vi "Render.vi"(9 "Size (1)":i32=1, 10 "Keys":map{string, string[]}(c390), 11 "Content in":string) -> (3 "Content out":string)   [LabVIEW 2021, in "HttpServer.lvlib"]
uses:
  HttpServer.lvlib
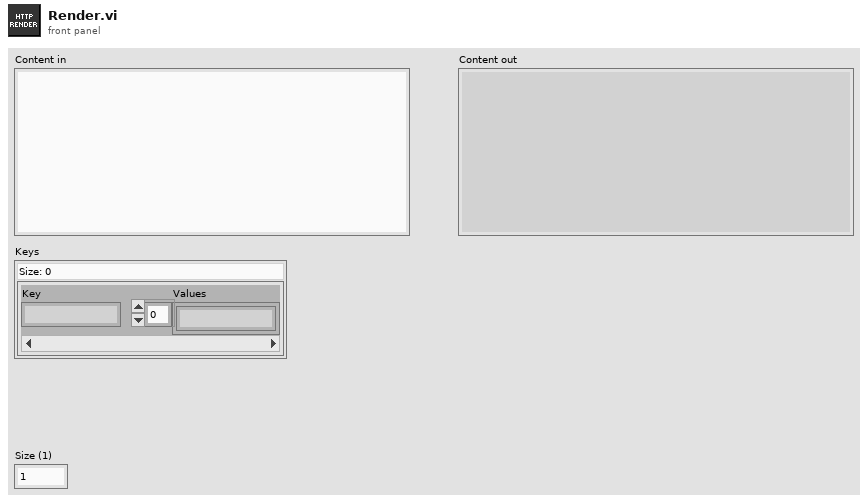
[diagram p1: front panel]
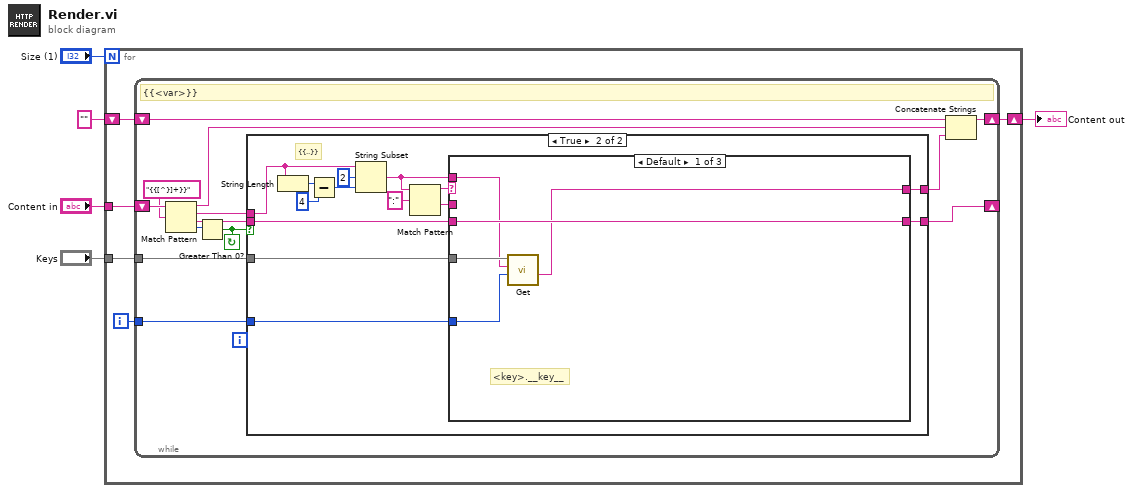
[diagram p0: block diagram]
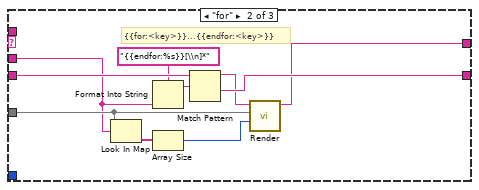
[diagram p3: hidden frame]
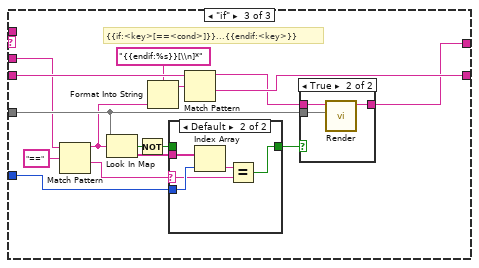
[diagram p4: hidden frame]
diagram:
  n1 = for {
    N: "Size (1)" -> [_]
    tunnel: "Keys" -> [w9]
    tunnel: "Content in" -> [w10]
    shift-right: [w8] -> w2
    shift-left: "" -> [w6]
    i -> [w7]
    n2 = while {
      shift-right: [w13] -> _
      shift-left: w10 -> [w23]
      shift-right: [w16] -> w8
      shift-left: w6 -> [w17]
      tunnel: w9 -> [w14]
      tunnel: w7 -> [w11]
      stop <- w20 continue-if-true
      # "{{<var>}}"
      n3 = Match Pattern(string=w23, regular expression="{{[^}]+}}") -> (before substring=w15:string, match substring=w19:string, after substring=w18:string, offset past match=w22:i32)  [unwired: 1 in]
      n4 = Greater Than 0?(x=w22) -> (x > 0?=w20:bool)
      n5 = case shown="True" w20 {
        tunnel: w19 -> [_ w37]
        tunnel: w18 -> [_ w29]
        tunnel: w14 -> [_ w27]
        tunnel: [_ w28] -> w13
        tunnel: [_ w26] -> w12
        tunnel: w11 -> [_ w25]
        frame False {
        }
        frame True {
          # "{{..}}"
          n6 = String Length(string=w37) -> (length=w36:i32)
          n7 = Subtract(x=w36, y=4) -> (x-y=w33:i32)
          n8 = String Subset(string=w37, offset (0)=2, length (rest)=w33) -> (substring=w24:string)
          n9 = Match Pattern(string=w24, regular expression=":") -> (before substring=w31:string, after substring=w30:string)  [unwired: 1 in, 2 out]
          n10 = case shown="Default" w31 {
            tunnel: w30 -> [_ w43 w59]
            tunnel: w29 -> [w42 w52 w68]
            tunnel: [w42 w49 w65] -> w28
            tunnel: w27 -> [w41 w47 w63]
            tunnel: [w38 w46 w62] -> w26
            tunnel: w25 -> [w39 _ w54]
            tunnel: w24 -> [w40 _ _]
            frame Default {
              # "<key>.__key__"
              n11 = call "Get.vi"("Idx (0)"=w39, "key"=w40, "Keys"=w41) -> ("Value out"=w38:string)  [unwired: 6 in, 2 out]
            }
            frame "for" {
              # "{{for:<key>}}...{{endfor:<key>}}"
              n12 = Look In Map(map=w47, key=w43) -> (value=w45:string[])  [unwired: 1 in, 1 out]
              n13 = Format Into String(format string="{{endfor:%s}}[\\n]*", w43) -> (resulting string=w50:string)  [unwired: 2 in, 1 out]
              n14 = Array Size(array=w45) -> (size(s)=w44:i32)
              n15 = Match Pattern(string=w52, regular expression=w50) -> (before substring=w48:string, after substring=w49:string)  [unwired: 1 in, 2 out]
              n16 = call "Render.vi"("Size (1)"=w44, "Keys"=w47, "Content in"=w48) -> ("Content out"=w46:string)  [unwired: 8 in]
            }
            frame "if" {
              # "{{if:<key>[==<cond>]}}...{{endif:<key>}}"
              n17 = Match Pattern(string=w59, regular expression="==") -> (before substring=w58:string, after substring=w57:string)  [unwired: 1 in, 2 out]
              n18 = Look In Map(map=w63, key=w58) -> (key not found?=w56:bool, value=w61:string[])  [unwired: 1 in]
              n19 = Not(x=w56) -> (.not. x?=w53:bool)
              n20 = Format Into String(format string="{{endif:%s}}[\\n]*", w58) -> (resulting string=w66:string)  [unwired: 2 in, 1 out]
              n21 = case shown="Default" w57 {
                selector: w57 -> [_ w71]
                tunnel: w61 -> [_ w74]
                tunnel: [w69 w70] -> w55
                tunnel: w53 -> [w69 _]
                tunnel: w54 -> [_ w73]
                frame "" {
                }
                frame Default {
                  n22 = Index Array(array=w74, index=w73) -> (element=w72:string)
                  n23 = Equal?(x=w72, y=w71) -> (x = y?=w70:bool)
                }
              }
              n24 = Match Pattern(string=w68, regular expression=w66) -> (before substring=w64:string, after substring=w65:string)  [unwired: 1 in, 2 out]
              n25 = case shown="True" w55 {
                tunnel: w64 -> [_ w77]
                tunnel: w63 -> [_ w76]
                tunnel: [_ w75] -> w62
                frame False {
                }
                frame True {
                  n26 = call "Render.vi"("Keys"=w76, "Content in"=w77) -> ("Content out"=w75:string)  [unwired: 9 in]
                }
              }
            }
          }
        }
      }
      n27 = Concatenate Strings(w17, w15, w12) -> (w16:string)
    }
  }
  "Content out" <- w2
